vi "current time string in ms.vi"(11 "ms to add":i64) -> (3 "time string in ms":string)   [LabVIEW 2020]
panel:
  out "time stamp":timestamp
  out "current time":timestamp
  out "double precision float":dbl format="%#_14f"
  out "time string":string
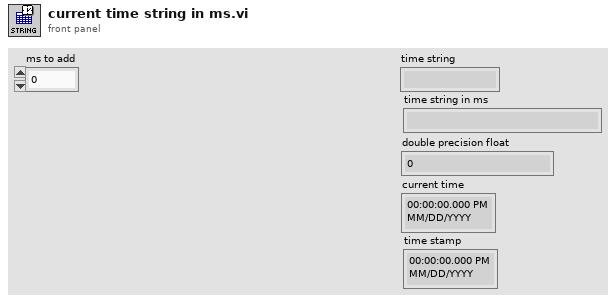
[diagram p1: front panel]
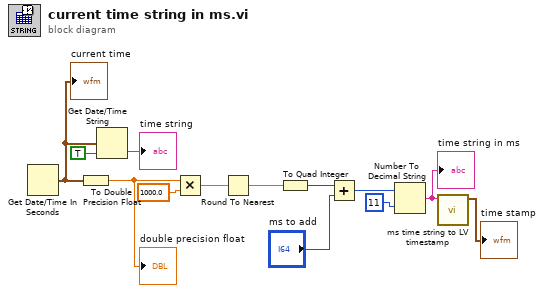
[diagram p0: block diagram]
diagram:
  n1 = Get Date/Time In Seconds() -> (seconds since 1Jan1904=w11:timestamp)
  "current time" <- w11
  n2 = To Double Precision Float(number=w11) -> (double precision float=w10:dbl)
  "double precision float" <- w10
  n3 = Get Date/Time String(seconds (now)=w11, want seconds? (F)=TRUE) -> (time string=→"time string":string)  [unwired: 1 in, 1 out]
  n4 = Multiply(x=w10, y=1000.0) -> (x*y=w8:dbl)
  n5 = Round To Nearest(number=w8) -> (nearest integer value=w6:dbl)
  n6 = To Quad Integer(1:w6) -> (0:w3:i64)
  n7 = Add(x=w3, y="ms to add") -> (x+y=w1:i64)
  n8 = Number To Decimal String(number=w1, width (-)=i16 11) -> (decimal integer string=w5:string)
  "time string in ms" <- w5
  n9 = call "ms time string to LV timestamp.vi"("String"=w5) -> ("Time Stamp"=→"time stamp":timestamp)  [unwired: 10 in]
